vi "CHECK_DEVICES_BUSY.vi"(7 "LabVIEW Web Service Request":refnum<class "Web Request.lvclass">, 11 "DEVICE_SN":string) -> (2 "Response":T1)   [LabVIEW 2015]
uses:
  <vilib>/wsapi/Web Request.lvclass
  Share Data/uPower_kit.ctl
panel:
  # "Use the Web Service Request input terminal to call the VIs on the Web Services palette. Do not remove it from the connector pane unless you don't need access to the palette."
  # "Each additional control wired to the connector pane will be available as an input in the URL. To include an indicator in terminal-mode output (the default setting), it must also be wired to the connector pane."
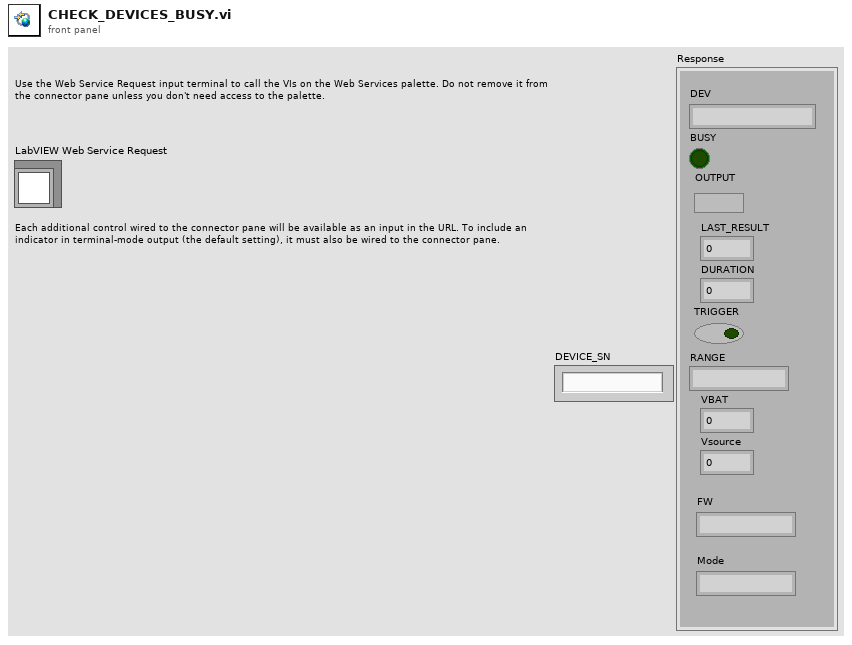
[diagram p1: front panel]
types:
  T1 = typedef "uPower_kit.ctl" = cluster{"DEV":string, "BUSY":bool, "VBAT":dbl, "OUTPUT":bool, "LAST_RESULT":dbl, "DURATION":u16, "TRIGGER":bool, "RANGE":string, "Vsource":dbl, "FW":string, "Mode":string}
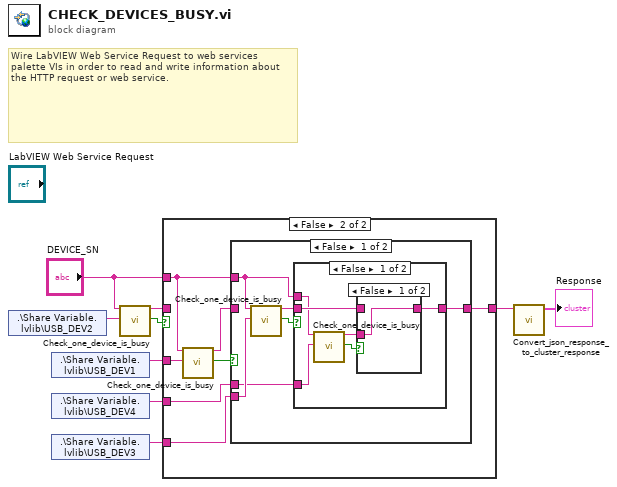
[diagram p0: block diagram]
diagram:
  # "Wire LabVIEW Web Service Request to web services palette VIs in order to read and write information about the HTTP request or web service."
  n1 = shared-variable ".\\Share Variable.lvlib\\USB_DEV2"() -> (w8:string)  [unwired: 1 in, 1 out]
  n2 = shared-variable ".\\Share Variable.lvlib\\USB_DEV1"() -> (w9:string)  [unwired: 1 in, 1 out]
  n3 = shared-variable ".\\Share Variable.lvlib\\USB_DEV4"() -> (w1:string)  [unwired: 1 in, 1 out]
  n4 = shared-variable ".\\Share Variable.lvlib\\USB_DEV3"() -> (w2:string)  [unwired: 1 in, 1 out]
  n5 = call "Check_one_device_is_busy.vi"("DEVICE_SN"="DEVICE_SN", "USB_DEV_json"=w8) -> ("USB_DEV_Json"=w6:string, "Device?"=w7:bool)  [unwired: 16 in]
  n6 = case shown="False" w7 {
    tunnel: w9 -> [_ w17]
    tunnel: "DEVICE_SN" -> [_ w13]
    tunnel: [w10 w14] -> w3
    tunnel: w6 -> [w10 _]
    tunnel: w2 -> [_ w12]
    tunnel: w1 -> [_ w11]
    frame True {
    }
    frame False {
      n7 = call "Check_one_device_is_busy.vi"("DEVICE_SN"=w13, "USB_DEV_json"=w17) -> ("USB_DEV_Json"=w15:string, "Device?"=w16:bool)  [unwired: 16 in]
      n8 = case shown="False" w16 {
        tunnel: w15 -> [_ w33]
        tunnel: [w21 w33] -> w14
        tunnel: w13 -> [w20 _]
        tunnel: w12 -> [w22 _]
        tunnel: w11 -> [w19 _]
        frame False {
          n9 = call "Check_one_device_is_busy.vi"("DEVICE_SN"=w20, "USB_DEV_json"=w22) -> ("USB_DEV_Json"=w18:string, "Device?"=w23:bool)  [unwired: 16 in]
          n10 = case shown="False" w23 {
            tunnel: w18 -> [w27 w32]
            tunnel: [w24 w32] -> w21
            tunnel: w20 -> [w26 _]
            tunnel: w19 -> [w25 _]
            frame False {
              n11 = call "Check_one_device_is_busy.vi"("DEVICE_SN"=w26, "USB_DEV_json"=w25) -> ("USB_DEV_Json"=w28:string, "Device?"=w29:bool)  [unwired: 16 in]
              n12 = case shown="False" w29 {
                tunnel: w28 -> [w30 w31]
                tunnel: w27 -> [_ _]
                tunnel: [w30 w31] -> w24
                frame False {
                }
                frame True {
                }
              }
            }
            frame True {
            }
          }
        }
        frame True {
        }
      }
    }
  }
  n13 = call "Convert_json_response_to_cluster_response.vi"("Json_Response_in"=w3) -> ("Response"=→"Response":T1)  [unwired: 10 in]
